vi "Table Column Reordering.vi"() -> ()   [LabVIEW 2016]
panel:
  out "Source Column":i32
  out "Destination Column":i32
  in  "Table Control":string[][](table)
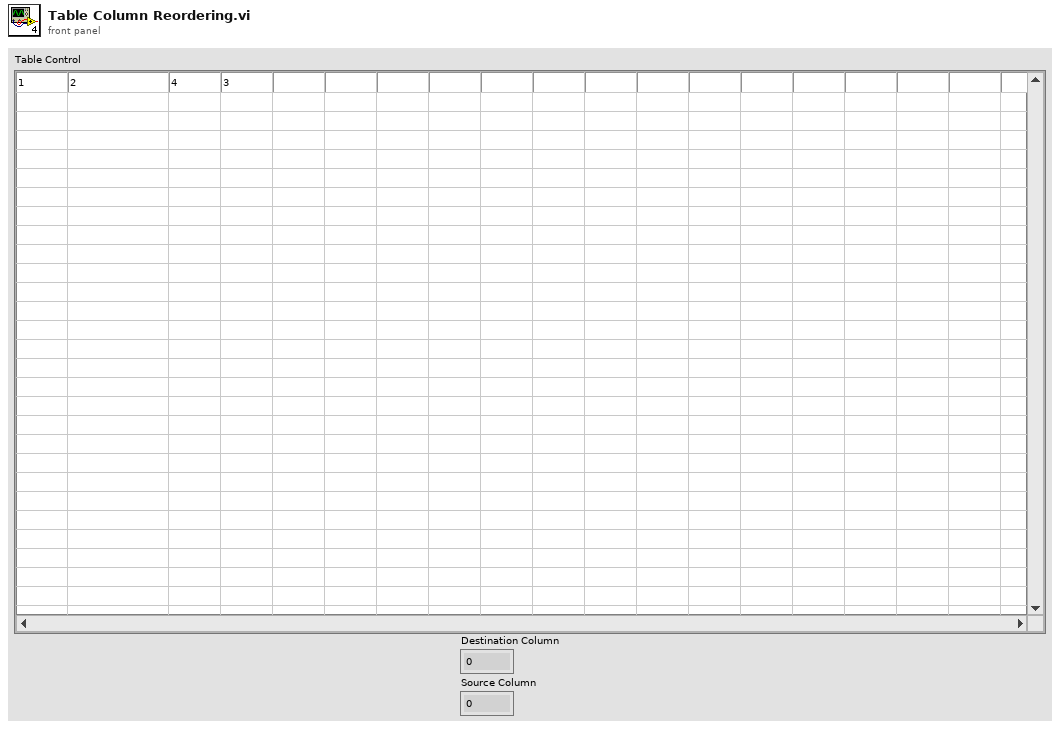
[diagram p1: front panel]
types:
  T1 = typedef "LVPoint32TypeDef.ctl" = cluster{"Horizontal":i32, "Vertical":i32}
  T2 = typedef "LVRowAndColumnTypeDef.ctl" = cluster{"Row":i32, "Column":i32}
  T3 = cluster{"data name":string, "drag data":variant}[]
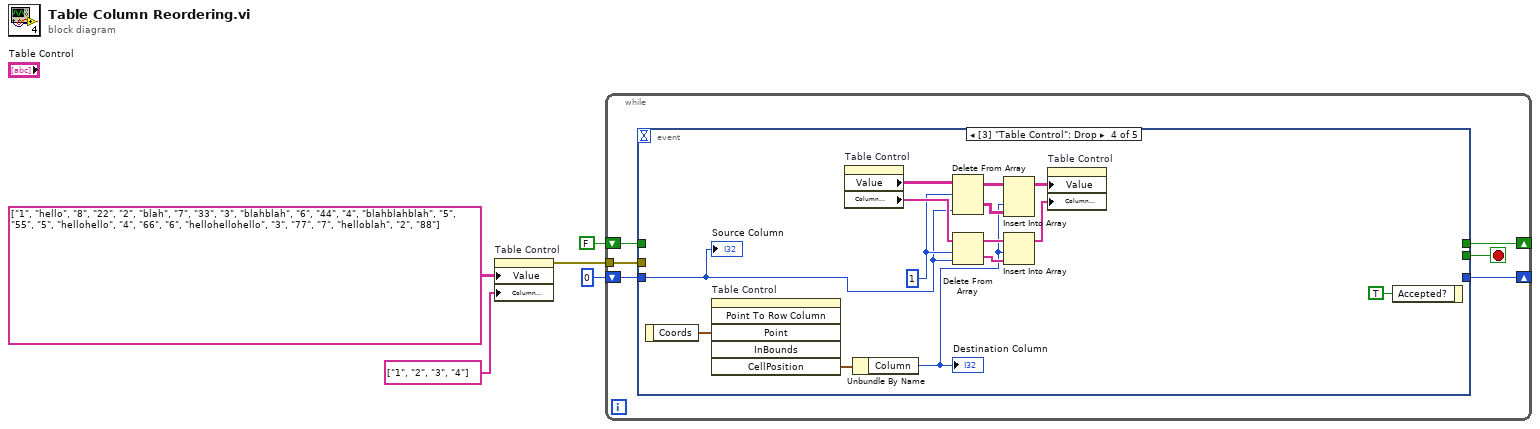
[diagram p0: block diagram]
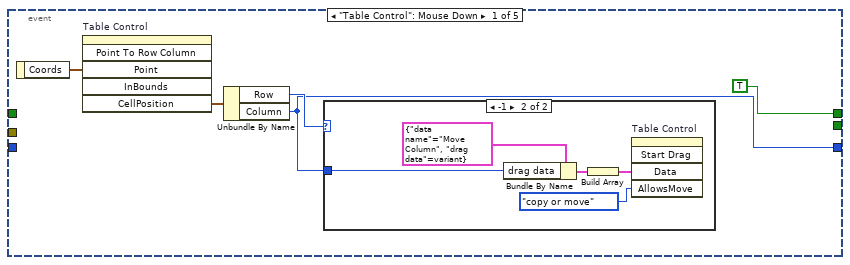
[diagram p2: hidden frame]
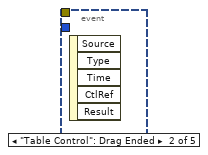
[diagram p4: hidden frame]
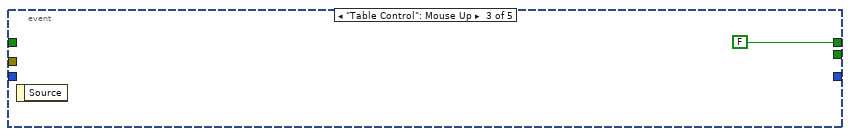
[diagram p5: hidden frame]
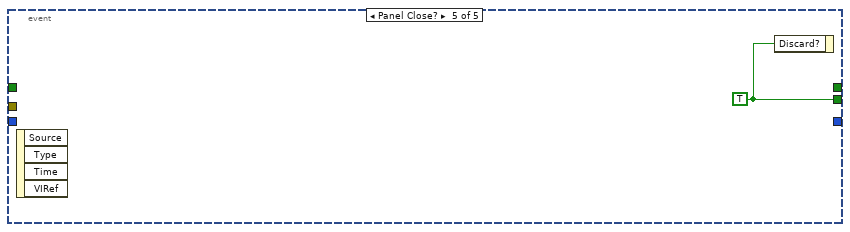
[diagram p6: hidden frame]
diagram:
  n1 = property on="Table Control" class="Tbl (strict)"("Value"=string[][] [["1", "hello", "8", "22"], ["2", "blah", "7", "33"], ["3", "blahblah", "6", "44"], ["4", "blahblahblah", "5", "55"], ["5", "hellohello", "4", "66"], ["6", "hellohellohello", "3", "77"], ["7", "helloblah", "2", "88"]] ("Table Control"), "Column Headers[]"=string[] ["1", "2", "3", "4"] ("Column Header Strings[]")) -> (error out=w2:errorcluster)  [unwired: 2 in, 1 out]
  n2 = while {
    shift-right: [w10] -> _
    shift-left: FALSE -> [w11]
    tunnel: w2 -> [w9]
    shift-right: [w7] -> _
    shift-left: 0 ("Column") -> [w6]
    stop <- w8 stop-if-true
    n3 = event shown="[3] \"Table Control\": Drop" {
      selector: _ -> [_ _ _ _ _]
      dyn-events: _ -> [_ _ _ _ _]
      timeout: _ -> [_ _ _ _ _]
      tunnel: w11 -> [_ _ _ _ _]
      tunnel: [TRUE _ FALSE _ _] -> w10
      tunnel: w9 -> [_ _ _ _ _]
      tunnel: [_ _ _ _ w37] -> w8
      tunnel: [w12 _ _ _ _] -> w7
      tunnel: w6 -> [_ _ _ w28 _]
      event "Table Control": Mouse Down {
        n4 = event-data() -> ("Coords"=w15:T1)  [unwired: 1 in]
        n5 = invoke on="Table Control" class="Tbl (strict)" method="Point To Row Column"("Point"=w15) -> ("CellPosition"=w14:T2)  [unwired: 5 in, 5 out]
        n6 = Unbundle By Name(w14) -> ("Row"=w13:i32, "Column"=w12:i32)
        n7 = case shown="-1" w13 {
          tunnel: w12 -> [_ w20]
          frame Default {
          }
          frame -1 {
            n8 = Bundle By Name(cluster=cluster{"data name":string, "drag data":variant} {"data name"="Move Column", "drag data"=variant}, "drag data"=w20) -> (w19:cluster{"data name":string, "drag data":variant})
            n9 = Build Array(w19) -> (w18:T3)
            n10 = invoke on="Table Control" class="Tbl (strict)" method="Start Drag"("Data"=w18, "AllowsMove"=enum32{"copy or move", "copy only", "move only"}."copy or move" ("Drag Mode")) -> ()  [unwired: 3 in, 5 out]
          }
        }
      }
      event "Table Control": Drag Ended {
        n11 = event-data() -> ()  [unwired: 1 in, 5 out]
      }
      event "Table Control": Mouse Up {
        n12 = event-data() -> ()  [unwired: 1 in, 1 out]
      }
      event "Table Control": Drop {
        w29 = 1 ("length")
        n13 = event-data() -> ("Coords"=w36:T1)  [unwired: 1 in]
        n14 = invoke on="Table Control" class="Tbl (strict)" method="Point To Row Column"("Point"=w36) -> ("CellPosition"=w35:T2)  [unwired: 5 in, 5 out]
        n15 = property on="Table Control" class="Tbl (strict)"() -> ("Value"=w34:string[][], "Column Headers[]"=w30:string[])  [unwired: 2 in, 2 out]
        n16 = Unbundle By Name(w35) -> ("Column"=w25:i32)
        "Destination Column" <- w25
        n17 = Delete From Array(array=w34, length=w29, index (col)=w28) -> (deleted portion=w32:string[][], array with subset deleted=w33:string[][])  [unwired: 1 in]
        n18 = Delete From Array(array=w30, length=w29, index=w28) -> (deleted portion=w26:string[], array with subset deleted=w27:string[])
        n19 = Insert Into Array(array=w33, index (col)=w25, new element=w32) -> (w31:string[][])  [unwired: 1 in]
        n20 = Insert Into Array(array=w27, index=w25, new element=w26) -> (w24:string[])
        n21 = property on="Table Control" class="Tbl (strict)"("Value"=w31, "Column Headers[]"=w24) -> ()  [unwired: 2 in, 2 out]
        n22 = event-data("Accepted?"=TRUE) -> ()  [unwired: 1 in, 1 out]
        "Source Column" <- w28
      }
      event Panel Close? {
        w37 = TRUE ("Discard?")
        n23 = event-data() -> ()  [unwired: 1 in, 4 out]
        n24 = event-data("Discard?"=w37) -> ()  [unwired: 1 in, 1 out]
      }
    }
  }
